vi "HTML Report Set Font Format.vi"(2 "Error In":errorcluster, 3 "Text Color (unchanged)":u32(colorbox)=16777216, 4 "Text Options":T1, 5 "Font Settings":T2={"Charset (-1)"=-1, "Weight (-1)"=-1, "Name"="", "Size"=" "}) -> (0 "error out":errorcluster, 1 "HTML formatting text":string)   [LabVIEW 2017, in "NI_ReportGenerationCore.lvlib"]
doc: "This VI creates the font face and color tags for HTML documents. It also creates option tags for text such as underline, bold, etc.\n\nThe Charset (-1) and Weight (-1) don't do anything."
uses:
  <vilib>/Utility/NIReport.llb/NI_ReportGenerationCore.lvlib
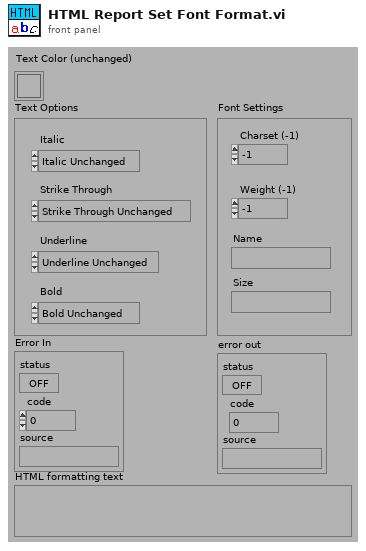
[diagram p1: front panel]
types:
  T1 = cluster{"Italic":enum16{"Italic Unchanged", "Italic On", "Italic Off"}, "Strike Through":enum16{"Strike Through Unchanged", "Strike Through On", "Strike Through Off"}, "Underline":enum16{"Underline Unchanged", "Underline On", "Underline Off"}, "Bold":enum16{"Bold Unchanged", "Bold On", "Bold Off"}}
  T2 = cluster{"Charset (-1)":i16, "Weight (-1)":i16, "Name":string, "Size":string}
  T3 = enum16{"Italic Unchanged", "Italic On", "Italic Off"}
  T4 = enum16{"Strike Through Unchanged", "Strike Through On", "Strike Through Off"}
  T5 = enum16{"Underline Unchanged", "Underline On", "Underline Off"}
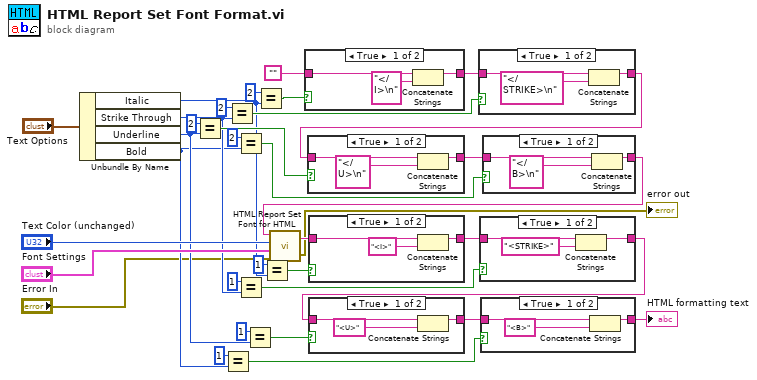
[diagram p0: block diagram]
diagram:
  n1 = Unbundle By Name("Text Options") -> ("Italic"=w13:T3, "Strike Through"=w11:T4, "Underline"=w9:T5, "Bold"=w6:enum16{"Bold Unchanged", "Bold On", "Bold Off"})
  n2 = Equal?(x=2, y=w9) -> (x = y?=w21:bool)
  n3 = Equal?(x=1, y=w6) -> (x = y?=w7:bool)
  n4 = Equal?(x=2, y=w11) -> (x = y?=w22:bool)
  n5 = Equal?(x=2, y=w6) -> (x = y?=w19:bool)
  n6 = Equal?(x=1, y=w11) -> (x = y?=w10:bool)
  n7 = Equal?(x=1, y=w9) -> (x = y?=w8:bool)
  n8 = Equal?(x=2, y=w13) -> (x = y?=w25:bool)
  n9 = Equal?(x=1, y=w13) -> (x = y?=w12:bool)
  n10 = case shown="True" w25 {
    tunnel: "" ("Substring") -> [w38 w39]
    tunnel: [w36 w39] -> w33
    frame True {
      n11 = Concatenate Strings(w38, "</I>\n") -> (w36:string)
    }
    frame False {
    }
  }
  n12 = case shown="True" w22 {
    tunnel: w33 -> [w42 w43]
    tunnel: [w40 w43] -> w32
    frame True {
      n13 = Concatenate Strings(w42, "</STRIKE>\n") -> (w40:string)
    }
    frame False {
    }
  }
  n14 = case shown="True" w21 {
    tunnel: w32 -> [w46 w47]
    tunnel: [w44 w47] -> w31
    frame True {
      n15 = Concatenate Strings(w46, "</U>\n") -> (w44:string)
    }
    frame False {
    }
  }
  n16 = case shown="True" w19 {
    tunnel: w31 -> [w50 w51]
    tunnel: [w48 w51] -> w4
    frame True {
      n17 = Concatenate Strings(w50, "</B>\n") -> (w48:string)
    }
    frame False {
    }
  }
  n18 = call <vilib>:"HTML Report Set Font for HTML.vi"("error in (no error)"="Error In", "Font Settings"="Font Settings", "Text Color (unchanged)"="Text Color (unchanged)", "HTML in"=w4) -> ("error out"=→"error out":errorcluster, "HTML w Font Setting"=w3:string)
  n19 = case shown="True" w12 {
    tunnel: w3 -> [w54 w55]
    tunnel: [w52 w55] -> w30
    frame True {
      n20 = Concatenate Strings(w54, "<I>") -> (w52:string)
    }
    frame False {
    }
  }
  n21 = case shown="True" w10 {
    tunnel: w30 -> [w58 w59]
    tunnel: [w56 w59] -> w29
    frame True {
      n22 = Concatenate Strings(w58, "<STRIKE>") -> (w56:string)
    }
    frame False {
    }
  }
  n23 = case shown="True" w8 {
    tunnel: w29 -> [w62 w63]
    tunnel: [w60 w63] -> w28
    frame True {
      n24 = Concatenate Strings(w62, "<U>") -> (w60:string)
    }
    frame False {
    }
  }
  n25 = case shown="True" w7 {
    tunnel: w28 -> [w66 w67]
    tunnel: [w64 w67] -> w18
    frame True {
      n26 = Concatenate Strings(w66, "<B>") -> (w64:string)
    }
    frame False {
    }
  }
  "HTML formatting text" <- w18
